vi "OpenFile.vi"(6 "operation (0:open)":T1(ring), 8 "error in (no error)":errorcluster, 9 "access (0:read/write)":enum16{"read/write", "read-only", "write-only"}(ring), 10 "File Path":path) -> (0 "error out":errorcluster, 3 "File out":refnum<class "File.lvclass">)   [LabVIEW 2021, in "File.lvclass"]
uses:
  File.lvclass
  File.lvclass/File.ctl
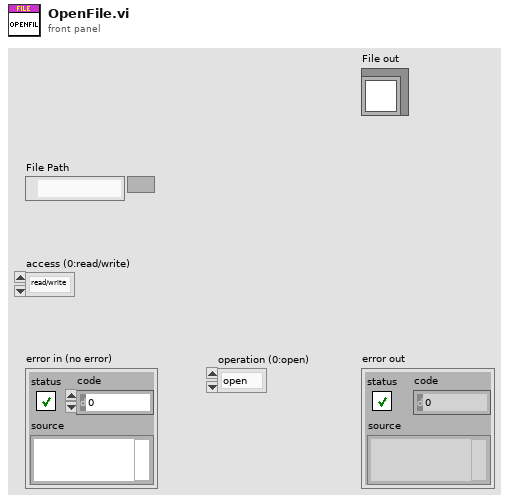
[diagram p1: front panel]
types:
  T1 = enum16{"open", "replace", "create", "open or create", "replace or create", "replace or create with confirmation"}
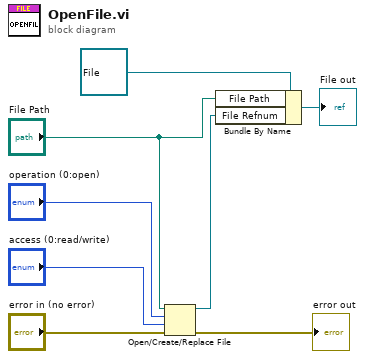
[diagram p0: block diagram]
diagram:
  n1 = Open/Create/Replace File(file path (use dialog)="File Path", error in="error in (no error)", operation (0:open)="operation (0:open)", access (0:read/write)="access (0:read/write)") -> (refnum out=w1:refnum<file>, error out=→"error out":errorcluster)  [unwired: 2 in, 1 out]
  n2 = Bundle By Name(cluster=refnum<class "File.lvclass"> refnum ("File in"), "File Path"="File Path", "File Refnum"=w1) -> (→"File out":refnum<class "File.lvclass">)
